vi "Button Toggle.vi"(10 "Input":bool) -> (2 "Output":bool)   [LabVIEW 2014]
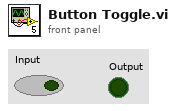
[diagram p1: front panel]
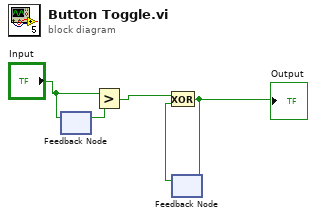
[diagram p0: block diagram]
diagram:
  n1 = feedback-in #1("Input") -> ()
  n2 = feedback #1() -> (w2:bool)  [unwired: 1 in]
  n3 = Greater?(x="Input", y=w2) -> (0:w3:bool)
  n4 = feedback #2() -> (w5:bool)  [unwired: 1 in]
  n5 = Exclusive Or(1:w5, 2:w3) -> (0:w4:bool)
  "Output" <- w4
  n6 = feedback-in #2(w4) -> ()
